vi "Format Operator Report.vi"(1 "Acceptable Measurement":bool) -> (0 "Operator Report":string)   [LabVIEW 2016]
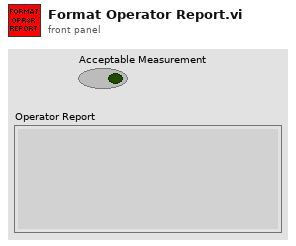
[diagram p1: front panel]
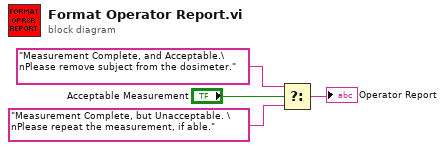
[diagram p0: block diagram]
diagram:
  n1 = Select(t="Measurement Complete, and Acceptable.\nPlease remove subject from the dosimeter.", s="Acceptable Measurement", f="Measurement Complete, but Unacceptable. \nPlease repeat the measurement, if able.") -> (s? t:f=→"Operator Report":string)
